vi "traffic_signal.vi"() -> ()   [LabVIEW 2019]
panel:
  out "Boolean 4":bool
  in  "stop":bool
  out "Boolean 3":bool
  out "Boolean 2":bool
  out "Boolean":bool
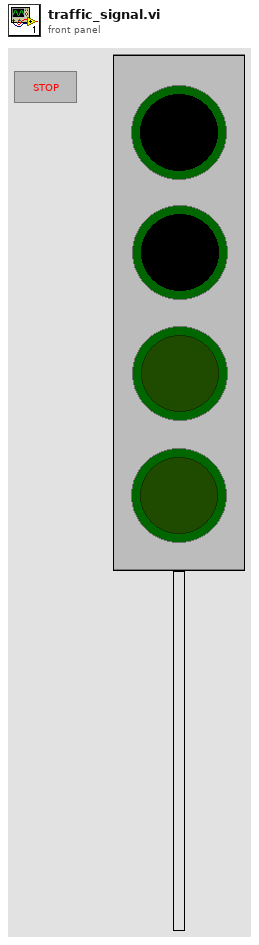
[diagram p1: front panel]
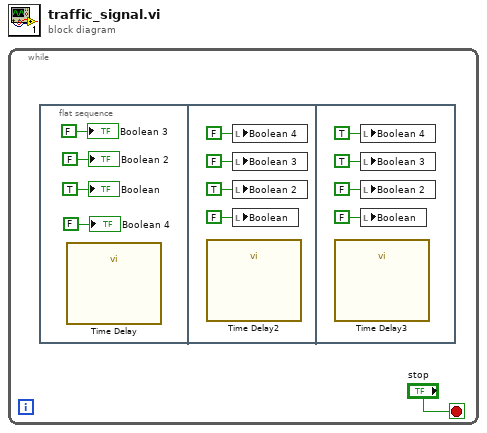
[diagram p0: block diagram]
diagram:
  n1 = while {
    stop <- "stop" stop-if-true
    n2 = flat-sequence {
      frame #0 {
        n3 = call "Time Delay"() -> ()  [unwired: 11 in, 1 out]
        "Boolean" <- TRUE
        "Boolean 2" <- FALSE
        "Boolean 3" <- FALSE
        "Boolean 4" <- FALSE
      }
      frame #1 {
        n4 = call "Time Delay2"() -> ()  [unwired: 11 in, 1 out]
        n5 = local write "Boolean 4"(FALSE) -> ()
        n6 = local write "Boolean 3"(FALSE) -> ()
        n7 = local write "Boolean 2"(TRUE) -> ()
        n8 = local write "Boolean"(FALSE) -> ()
      }
      frame #2 {
        n9 = call "Time Delay3"() -> ()  [unwired: 11 in, 1 out]
        n10 = local write "Boolean 4"(TRUE) -> ()
        n11 = local write "Boolean 3"(TRUE) -> ()
        n12 = local write "Boolean 2"(FALSE) -> ()
        n13 = local write "Boolean"(FALSE) -> ()
      }
    }
  }
